vi "_PC_RTLoop_ReadCurrentMSEvent.vi"(7 "Function":enum16{"Init", "Get Data", "Close"}(ring)=enum."Get Data", 8 "error in (no error)":errorcluster, 10 "connect?":bool, 11 "Firmware string refin":refnum<vi>) -> (0 "error out":errorcluster)   [LabVIEW 2018]
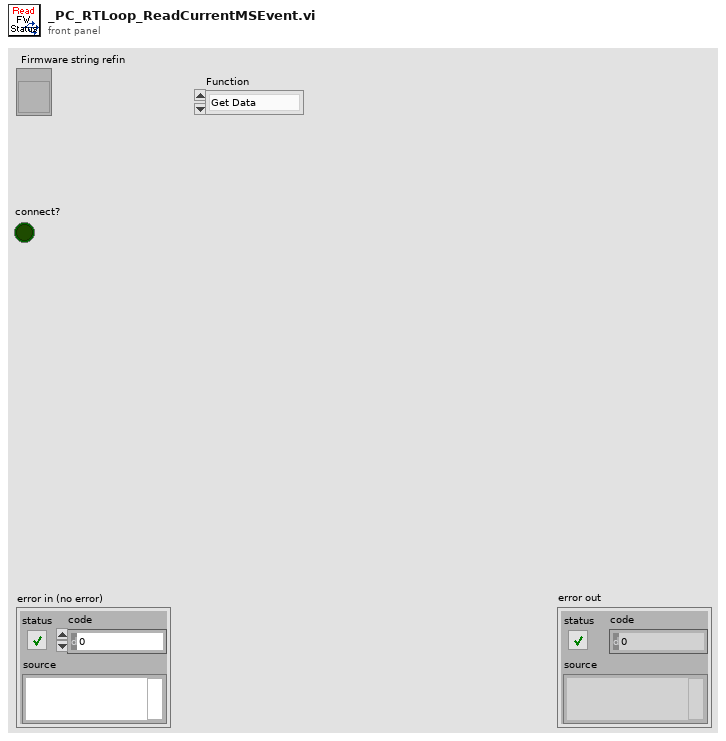
[diagram p1: front panel]
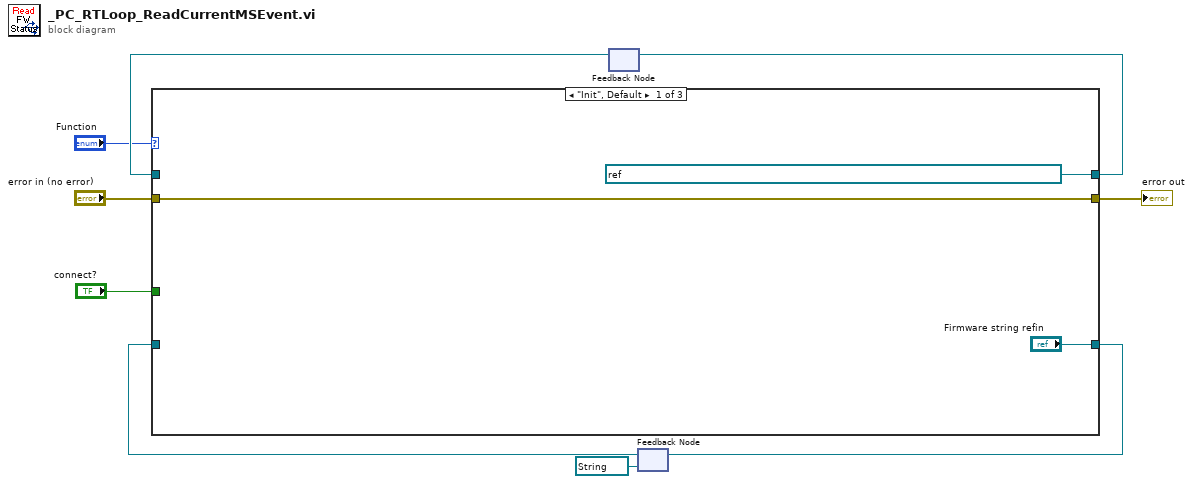
[diagram p0: block diagram]
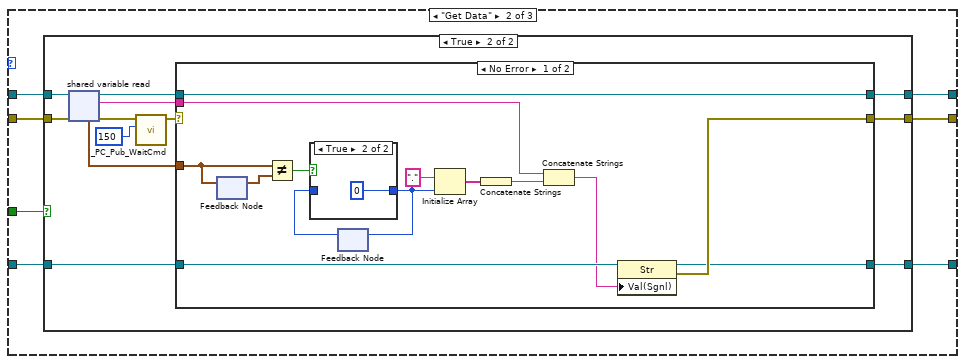
[diagram p2: hidden frame]
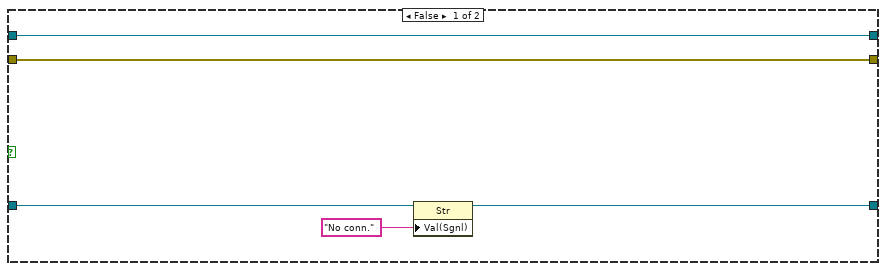
[diagram p3: hidden frame]
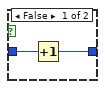
[diagram p4: hidden frame]
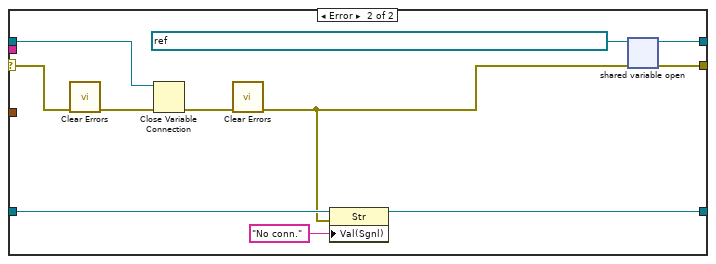
[diagram p5: hidden frame]
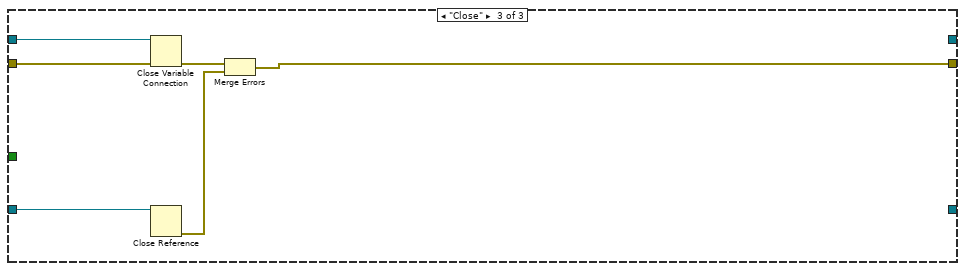
[diagram p6: hidden frame]
diagram:
  n1 = feedback #1() -> (w8:refnum<k21>)  [unwired: 1 in]
  n2 = feedback #2(refnum<vi> refnum ("Firmware string refin")) -> (w6:refnum<vi>)
  n3 = case shown="\"Init\", Default" "Function" {
    tunnel: w8 -> [_ w19 w70]
    tunnel: [refnum<k21> "ni.var.psp://NI-sbRIO/_RT_CtrlLoop_MassAnalysing_Variable/FirmwareStatus" ("shared variable refnum in") w18 _] -> w9
    tunnel: ["Firmware string refin" w15 _] -> w7
    tunnel: w6 -> [_ w16 w68]
    tunnel: [w10 w17 w65] -> w4
    tunnel: "error in (no error)" -> [w10 w14 w69]
    tunnel: "connect?" -> [_ w13 _]
    frame "Init", Default {
    }
    frame "Get Data" {
      n4 = case shown="True" w13 {
        tunnel: w19 -> [w21 w36]
        tunnel: [w21 w34] -> w18
        tunnel: [w20 w33] -> w17
        tunnel: w16 -> [w24 w30]
        tunnel: [w22 w29] -> w15
        tunnel: w14 -> [w20 w28]
        frame False {
          n5 = property class="Str"(reference=w24, "Val(Sgnl)"="No conn." ("t")) -> (reference out=w22:refnum<vi>)  [unwired: 1 in, 1 out]
        }
        frame True {
          n6 = shared-variable-read(w36, w28) -> (w35:refnum<k21>, w27:errorcluster, w32:string, w31:timestamp)
          n7 = call "_PC_Pub_WaitCmd.vi"("milliseconds to wait"=u32 150, "error in (no error)"=w27) -> ("error out"=w26:errorcluster)  [unwired: 9 in]
          n8 = case shown="No Error" w26 {
            selector: w26 -> [_ w56]
            tunnel: w35 -> [w50 w64]
            tunnel: [w50 w63] -> w34
            tunnel: [w38 w60] -> w33
            tunnel: w32 -> [w42 _]
            tunnel: w31 -> [w43 _]
            tunnel: w30 -> [w40 w59]
            tunnel: [w37 w58] -> w29
            frame No Error {
              n9 = feedback #3() -> (w49:timestamp)  [unwired: 1 in]
              n10 = feedback-in #3(w43) -> ()
              n11 = Not Equal?(x=w43, y=w49) -> (x != y?=w48:bool)
              n12 = feedback #4() -> (w47:i32)  [unwired: 1 in]
              n13 = case shown="True" w48 {
                tunnel: [w51 0] -> w45
                tunnel: w47 -> [w52 _]
                frame False {
                  n14 = Increment(x=w52) -> (x+1=w51:i32)
                }
                frame True {
                }
              }
              n15 = feedback-in #4(w45) -> ()
              n16 = Initialize Array(".", w45) -> (w44:string[])
              n17 = Concatenate Strings(w44) -> (w41:string)
              n18 = Concatenate Strings(w42, w41) -> (w39:string)
              n19 = property class="Str"(reference=w40, "Val(Sgnl)"=w39) -> (reference out=w37:refnum<vi>, error out=w38:errorcluster)  [unwired: 1 in]
            }
            frame Error {
              n20 = call <vilib>:"Clear Errors.vi"("error in (no error)"=w56) -> ("error out"=w55:errorcluster)  [unwired: 5 in, 1 out]
              n21 = Close Variable Connection(8:w55, 11:w64) -> (0:w61:errorcluster)
              n22 = call <vilib>:"Clear Errors.vi"("error in (no error)"=w61) -> ("error out"=w54:errorcluster)  [unwired: 5 in, 1 out]
              n23 = property class="Str"(reference=w59, error in=w54, "Val(Sgnl)"="No conn." ("t")) -> (reference out=w58:refnum<vi>)  [unwired: 1 out]
              n24 = shared-variable-open(refnum<k21> "ni.var.psp://NI-sbRIO/_RT_CtrlLoop_MassAnalysing_Variable/FirmwareStatus" ("shared variable refnum in"), w54) -> (w63:refnum<k21>, w60:errorcluster)
            }
          }
        }
      }
    }
    frame "Close" {
      n25 = Close Variable Connection(8:w69, 11:w70) -> (0:w66:errorcluster)
      n26 = Close Reference(reference=w68) -> (error out=w67:errorcluster)  [unwired: 1 in]
      n27 = Merge Errors(w66, w67) -> (w65:errorcluster)
    }
  }
  "error out" <- w4
  n28 = feedback-in #1(w9) -> ()
  n29 = feedback-in #2(w7) -> ()
